vi "Get Row Values.vi"(7 "Sheet Name":string, 8 "error in":errorcluster, 10 "Cell Addresses":string="A1:B1", 11 "SpreadsheetDoc in":refnum<k24>) -> (0 "error out":errorcluster, 1 "Types":T1[](array[typedef]), 2 "Cell Values":T2(array[cluster]) {"Time Stamp" format="%<%x %.3X>T"}, 3 "SpreadsheetDoc out":refnum<k24>)   [LabVIEW 2019, in "Open Xml.lvlib"]
uses:
  Open Xml.lvlib
  D:/git/Open-Xml-LabVIEW/Source/DocumentFormat.OpenXml.dll
  DocumentFormat.OpenXml.dll
  Cell DataType.ctl
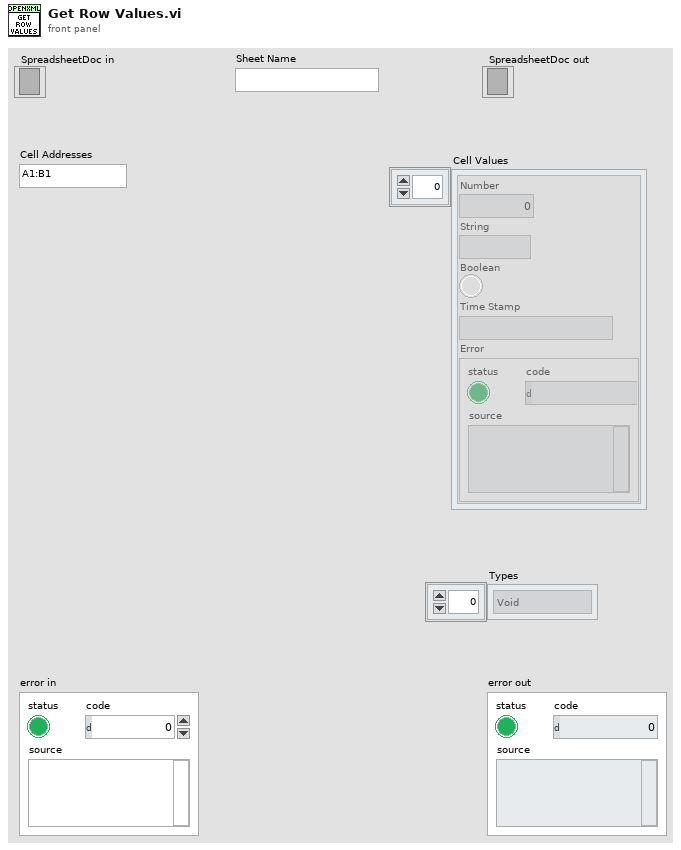
[diagram p1: front panel]
types:
  T1 = typedef "Open Xml.lvlib/Cell DataType.ctl" = enum16{"Void", "Boolean", "Number", "Error", "SharedString", "String", "InlineString", "Date"}
  T2 = cluster{"Number":dbl, "String":string, "Boolean":bool, "Time Stamp":timestamp, "Error":errorcluster}[]
  T3 = cluster{"Number":dbl, "String":string, "Boolean":bool, "Time Stamp":timestamp, "Error":errorcluster}
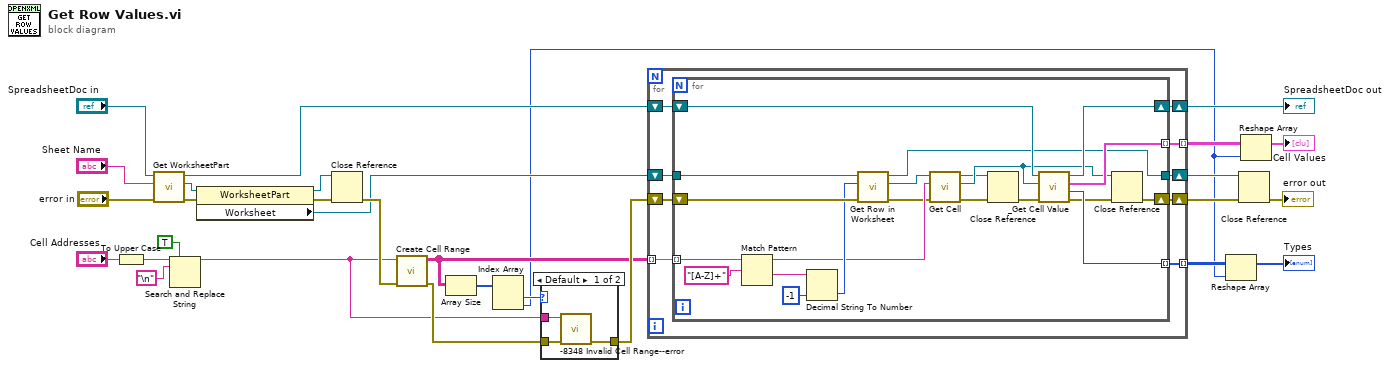
[diagram p0: block diagram]
diagram:
  n1 = To Upper Case(1:"Cell Addresses") -> (0:w19:string)
  n2 = call "Get WorksheetPart.vi"("error in"="error in", "Sheet Name"="Sheet Name", "SpreadsheetDocument in"="SpreadsheetDoc in") -> ("error out"=w15:errorcluster, "WorksheetPart"=w14:refnum<k24>, "SpreadsheetDocument out"=w24:refnum<k24>)  [unwired: 6 in]
  n3 = Search and Replace String(replace all?=TRUE ("replace all? (F)"), input string=w19, search string="\n") -> (result string=w5:string)  [unwired: 5 in, 3 out]
  n4 = property class="WorksheetPart"(reference=w14, error in=w15) -> (reference out=w11:refnum<k24>, error out=w13:errorcluster, "Worksheet"=w10:refnum<k24>)
  n5 = Close Reference(reference=w11, error in (no error)=w13) -> (error out=w12:errorcluster)
  n6 = call "Create Cell Range.vi"("error in"=w12, "Cell Range"=w5) -> ("error out"=w21:errorcluster, "Cell Range"=w8:string[][])  [unwired: 8 in]
  n7 = Array Size(array=w8) -> (size(s)=w7:i32[])
  n8 = Index Array(array=w7) -> (element #1=w6:i32, element #2=w1:i32)  [unwired: 2 in]
  n9 = case shown="Default" w6 {
    tunnel: w21 -> [w32 w33]
    tunnel: [w31 w33] -> w9
    tunnel: w5 -> [w30 _]
    frame Default {
      n10 = call "-8348 Invalid Cell Range--error.vi"("error in"=w32, "Argument"=w30) -> ("error out"=w31:errorcluster)  [unwired: 9 in]
    }
    frame 1 {
    }
  }
  n11 = for {
    tunnel: w8 -> [w40] mode=indexing
    tunnel: [w38] -> w3 mode=indexing
    tunnel: [w37] -> w23 mode=indexing
    shift-right: [w41] -> w27
    shift-left: w24 -> [w39]
    shift-right: [w42] -> w28
    shift-left: w9 -> [w35]
    shift-right: [w36] -> w22
    shift-left: w10 -> [w34]
    n12 = for {
      tunnel: [w58] -> w38 mode=indexing
      tunnel: [w57] -> w37 mode=indexing
      shift-right: [w61] -> w42
      shift-left: w35 -> [w62]
      shift-right: [w59] -> w41
      shift-left: w39 -> [w60]
      tunnel: w40 -> [w48] mode=indexing
      tunnel: [w46] -> w36
      tunnel: w34 -> [w43]
      n13 = Match Pattern(string=w48, regular expression="[A-Z]+") -> (after substring=w50:string)  [unwired: 1 in, 3 out]
      n14 = Decimal String To Number(string=w50, default (0L)=i64 -1 ("default (0 I32)")) -> (number=w49:i64)  [unwired: 1 in, 1 out]
      n15 = call "Get Row in Worksheet.vi"("error in"=w62, "RowIndex"=w49, "Worksheet in"=w43) -> ("error out"=w47:errorcluster, "Row out"=w45:refnum<k24>, "Worksheet out"=w46:refnum<k24>)  [unwired: 6 in]
      n16 = call "Get Cell.vi"("error in"=w47, "Cell Address"=w48, "Row in"=w45) -> ("error out"=w56:errorcluster, "Cell"=w53:refnum<k24>, "Row out"=w44:refnum<k24>)  [unwired: 6 in]
      n17 = Close Reference(reference=w44, error in (no error)=w56) -> (error out=w55:errorcluster)
      n18 = call "_Get Cell Value.vi"("error in"=w55, "Cell"=w53, "SpreadsheetDoc in"=w60) -> ("error out"=w54:errorcluster, "Type"=w57:T1, "Cell Value"=w58:T3, "SpreadsheetDocument out"=w59:refnum<k24>)  [unwired: 5 in]
      n19 = Close Reference(reference=w53, error in (no error)=w54) -> (error out=w61:errorcluster)
    }
  }
  "SpreadsheetDoc out" <- w27
  n20 = Reshape Array(w23, w1) -> (→"Types":T1[])
  n21 = Close Reference(reference=w22, error in (no error)=w28) -> (error out=→"error out":errorcluster)
  n22 = Reshape Array(w3, w1) -> (→"Cell Values":T2)
